vi "Sort User[ ].vi"(8 "error in (no error)":errorcluster, 11 "Telegram Class in":refnum<class "Telegram Class.lvclass">) -> (0 "error out":errorcluster, 3 "Telegram Class out":refnum<class "Telegram Class.lvclass">)   [LabVIEW 2015, in "Telegram Library.lvlib" / "Telegram Class.lvclass"]
doc: "Created IvanLis by LabVIEW Portal\nProfile: http://labviewportal.org/memberlist.php?mode=viewprofile&u=987\neMail: IvanLisanov@gMail.com\nTelegram: https://t.me/IvanLis"
uses:
  Telegram Class.lvclass
  Telegram Class.lvclass/Telegram Class.ctl
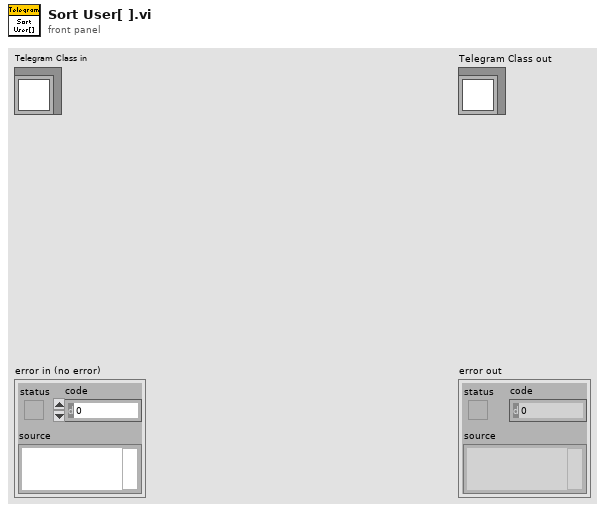
[diagram p1: front panel]
types:
  T1 = typedef "Telegram Library.lvlib/User.ctl" = cluster{"id":i64, "phone_number":string, "username":string, "last_name":string, "first_name":string}
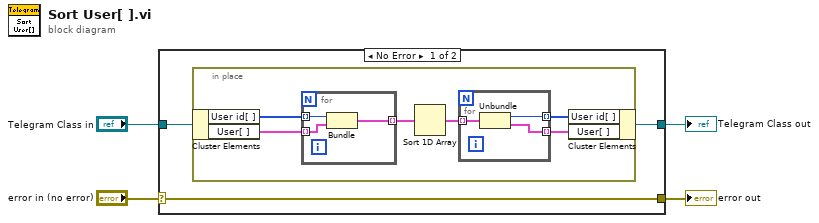
[diagram p0: block diagram]
diagram:
  n1 = case shown="No Error" "error in (no error)" {
    selector: "error in (no error)" -> [w7 w21]
    tunnel: [w7 w21] -> w3
    tunnel: [w5 w20] -> w1
    tunnel: "Telegram Class in" -> [w6 w20]
    frame No Error {
      n2 = in-place {
        n3 = in-place-cluster #1(w6) -> ("User id[ ]"=w13:i64[], "User[ ]"=w12:T1[])
        n4 = for {
          tunnel: w13 -> [w16] mode=indexing
          tunnel: w12 -> [w15] mode=indexing
          tunnel: [w14] -> w11 mode=indexing
          n5 = Bundle("id"=w16, "User"=w15) -> (w14:cluster{"id":i64, "User":T1})  [unwired: 1 in]
        }
        n6 = Sort 1D Array(array=w11) -> (sorted array=w10:cluster{"id":i64, "User":T1}[])
        n7 = for {
          tunnel: w10 -> [w19] mode=indexing
          tunnel: [w18] -> w9 mode=indexing
          tunnel: [w17] -> w8 mode=indexing
          n8 = Unbundle(w19) -> ("id"=w18:i64, "User"=w17:T1)
        }
        n9 = in-place-cluster #1("User id[ ]"=w9, "User[ ]"=w8) -> (w5:refnum<class "Telegram Class.lvclass">)
      }
    }
    frame Error {
    }
  }
  "error out" <- w3
  "Telegram Class out" <- w1
